vi "CIMAQ_Attenuate.vi"(5 "Mode":enum16{"Lowpass", "Highpass"}(ring), 6 "Cutoff (%)":dbl=5.0, 7 "error in (no error)":errorcluster, 9 "Image Dst":T1, 10 "Image Src":T1) -> (0 "error out":errorcluster, 3 "Image":T1(plugin-control))   [LabVIEW 2017]
uses:
  <vilib>/vision/Image Controls.llb/IMAQ Image.ctl
  <vilib>/Analysis/baseanly.llb/Quick Scale 2D.vi
  <vilib>/vision/NI_Vision_Development_Module.lvlib
  <vilib>/Analysis/NI_AALBase.lvlib
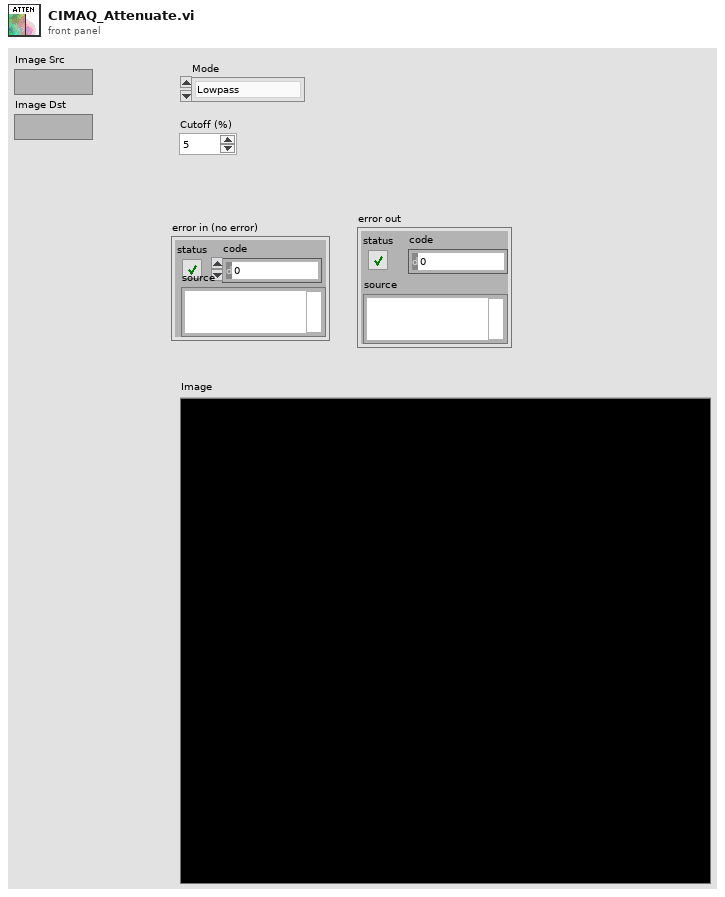
[diagram p1: front panel]
types:
  T1 = typedef "IMAQ Image.ctl" = refnum<image>
  T2 = typedef "Image Type" = u32
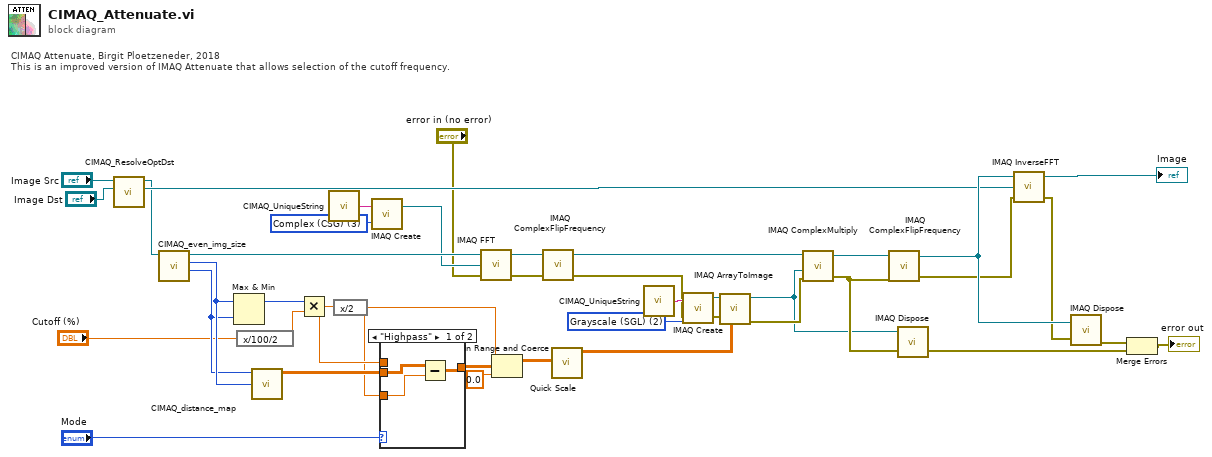
[diagram p0: block diagram]
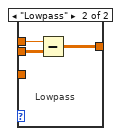
[diagram p2: hidden frame]
diagram:
  w30 = T2 2 items=["Grayscale (U8)", "Grayscale (I16)", "Grayscale (SGL)", "Complex (CSG)", "RGB (U32)", "HSL (U32)", "RGB (U64)", "Grayscale (U16)"] ("Image Type")
  w37 = T2 3 items=["Grayscale (U8)", "Grayscale (I16)", "Grayscale (SGL)", "Complex (CSG)", "RGB (U32)", "HSL (U32)", "RGB (U64)", "Grayscale (U16)"] ("Image Type")
  # "CIMAQ Attenuate, Birgit Ploetzeneder, 2018\nThis is an improved version of IMAQ Attenuate that allows selection of the cutoff frequency."
  n1 = call <userlib>:"CIMAQ_ResolveOptDst.vi"("Dst(optional)"="Image Dst", "Src"="Image Src") -> ("Dst"=w19:T1, "Src"=w17:T1)  [unwired: 7 in]
  n2 = call <userlib>:"CIMAQ_even_img_size.vi"("img"=w17) -> ("resolution_y"=w34:u32, "resolution_x"=w35:u32, "img"=w41:T1)  [unwired: 8 in]
  n3 = Max & Min(x=w35, y=w34) -> (max(x,y)=w32:u32)  [unwired: 1 out]
  n4 = expression code="x/100/2"("Cutoff (%)") -> (w33:dbl)
  n5 = call <userlib>:"CIMAQ_distance_map.vi"("size_x"=w35, "size_y"=w34) -> ("distance_map"=w27:dbl[][])  [unwired: 9 in]
  n6 = Multiply(x=w32, y=w33) -> (x*y=w4:dbl)
  n7 = call <userlib>:"CIMAQ_UniqueString.vi"() -> ("String"=w24:string)  [unwired: 5 in]
  n8 = expression code="x/2"(w4) -> (w3:dbl)
  n9 = call "IMAQ Create"("Image Name"=w24, "Image Type"=w37) -> ("New Image"=w36:T1)  [unwired: 3 in, 1 out]
  n10 = case shown="\"Highpass\"" "Mode" {
    tunnel: w27 -> [w44 w47]
    tunnel: [w43 w46] -> w26
    tunnel: w4 -> [_ w45]
    tunnel: w3 -> [w42 _]
    frame "Highpass" {
      n11 = Subtract(x=w44, y=w42) -> (x-y=w43:dbl[][])
    }
    frame "Lowpass" {
      # "Lowpass"
      n12 = Subtract(x=w45, y=w47) -> (x-y=w46:dbl[][])
    }
  }
  n13 = call "IMAQ FFT"("error in (no error)"="error in (no error)", "Image Dst"=w36, "Image Src"=w41) -> ("error out"=w14:errorcluster, "Image Dst Out"=w40:T1)  [unwired: 1 in]
  n14 = In Range and Coerce(upper limit=w3, x=w26, lower limit=0.0 ("x*y")) -> (coerced(x)=w25:dbl[][])  [unwired: 1 out]
  n15 = call "IMAQ ComplexFlipFrequency"("error in (no error)"=w14, "Image Src"=w40) -> ("error out"=w13:errorcluster, "Image Dst Out"=w39:T1)  [unwired: 2 in]
  n16 = call-poly <vilib>:"Quick Scale.vi"("X"=w25) -> ("Yij=Xij/Max|X|"=w16:dbl[][])  [unwired: 2 out]
  n17 = call <userlib>:"CIMAQ_UniqueString.vi"() -> ("String"=w23:string)  [unwired: 5 in]
  n18 = call "IMAQ Create"("Image Name"=w23, "Image Type"=w30, "error in (no error)"=w13) -> ("New Image"=w38:T1, "error out"=w12:errorcluster)  [unwired: 2 in]
  n19 = call "IMAQ ArrayToImage"("Image Pixels (Float)"=w16, "error in (no error)"=w12, "Image"=w38) -> ("error out"=w11:errorcluster, "Image Out"=w2:T1)  [unwired: 7 in]
  n20 = call "IMAQ ComplexMultiply"("Image Src A"=w39, "Image Src B"=w2, "error in (no error)"=w11) -> ("Image Dst Out"=w1:T1, "error out"=w10:errorcluster)  [unwired: 4 in]
  n21 = call "IMAQ ComplexFlipFrequency"("error in (no error)"=w10, "Image Src"=w1) -> ("error out"=w9:errorcluster, "Image Dst Out"=w22:T1)  [unwired: 2 in]
  n22 = call "IMAQ Dispose"("Image"=w2, "error in (no error)"=w10) -> ("error out"=w7:errorcluster)  [unwired: 4 in]
  n23 = call "IMAQ InverseFFT"("error in (no error)"=w9, "Image Dst"=w19, "Image Src"=w22) -> ("error out"=w21:errorcluster, "Image Dst Out"=→"Image":T1)  [unwired: 1 in]
  n24 = call "IMAQ Dispose"("Image"=w22, "error in (no error)"=w21) -> ("error out"=w8:errorcluster)  [unwired: 4 in]
  n25 = Merge Errors(w8, w7) -> (→"error out":errorcluster)
